vi "Uninit.vi"(8 "Error in":errorcluster, 11 "Base Actor in":refnum<class "Base Actor.lvclass">) -> (0 "Error out":errorcluster, 3 "Base Actor out":refnum<class "Base Actor.lvclass">)   [LabVIEW 2020, in "jettl.lvlib" / "Actor.lvlib" / "Base Actor.lvclass"]
uses:
  Base Actor.lvclass
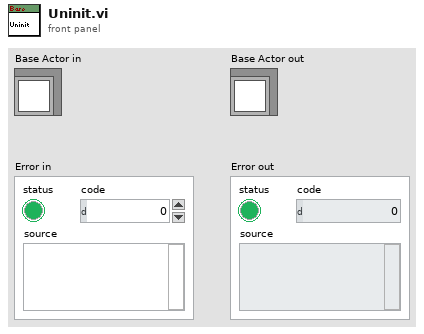
[diagram p1: front panel]
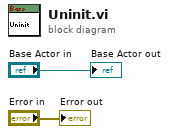
[diagram p0: block diagram]
diagram:
  "Base Actor out" <- "Base Actor in"
  "Error out" <- "Error in"
